vi "resourcesInquiry.vi"(8 "error in (no error)":errorcluster, 11 "HWController in":refnum<class "HWController.lvclass">) -> (0 "error out":errorcluster, 3 "HWController out":refnum<class "HWController.lvclass">)   [LabVIEW 2011, in "Hardware.lvlib" / "HWControllers.lvlib" / "HWController.lvclass"]
uses:
  HWController.lvclass
  HWController.lvclass/HWController.ctl
  HWControllerEvents/HWControllerEvents.lvclass
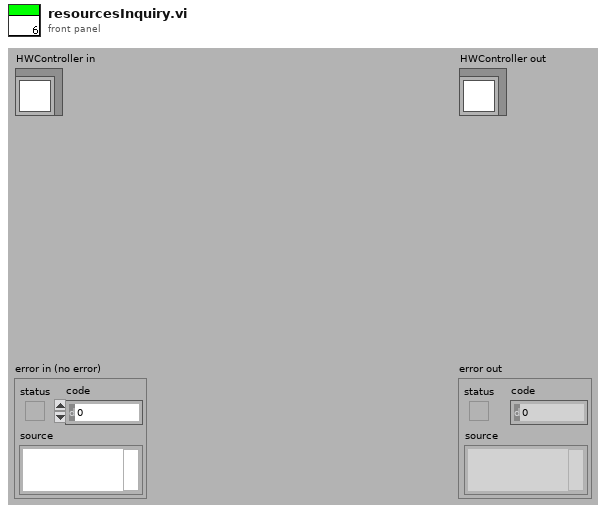
[diagram p1: front panel]
types:
  T1 = enum16{"start", "stop", "statusInquiry", "configure", "resetError", "resourcesInquiry", "reserveResources", "initialise", "resetAllChannels", "staticUpdate", "close", "HWStatus", "error", "resourcesAvailable", "resourcesReserved"}
  T2 = cluster{"incomingEventTypes":cluster{"start":cluster{"Boolean":bool}, "stop":cluster{"Boolean":bool}, "statusInquiry":cluster{"Boolean":bool}, "configure":cluster{"DPScriptPath":path, "TimeStamp":string, "HWLoop?":bool}, "resetError":cluster{"Boolean":bool}, "resourcesInquiry":cluster{"Boolean":bool}, "reserveResources":cluster{"HWList":string[]}, "initialise":cluster{"HWList":string[]}, "close":cluster{"Boolean":bool}, "resetAllChannels":cluster{"Boolean":bool}, "staticChannelUpdate":cluster{"channel_address":string, "calibratedValue":dbl}, "runScript":cluster{"DPScriptPath":path, "TimeStamp":string, "HWLoop?":bool}, "compilingScript":cluster{"Path":path}, "compiledScript":cluster{"Path":path, "timeCompileAt":string}, "compilerError":cluster{"Path":path}, "configureCompiledScript":cluster{"DPScriptPath":path, "TimeStamp":string, "HWLoop?":bool, "CompiledScript":cluster{"ScriptListCompiler.lvclass":refnum<class "ScriptListCompiler.lvclass">, "aoChannels":refnum<class "AnalogOutput.lvclass">[], "doChannels":refnum<class "DigitalOutput.lvclass">[], "rfChannels":refnum<class "DDSOutput.lvclass">[]}}, "restartCompiler":cluster{"restart":bool}, "staticRfChannelUpdate":cluster{"channel_address":string, "Output":cluster{"Frequency(MHz)":dbl, "Amplitude":dbl, "Phase":dbl, "OutputForm":enum16{"Sine", "Square", "Triangle", "Arbitrary"}}}, "cameraUpdate":cluster{"Camera":string, "Type":string, "settings":path}}, "outgoingEventTypes":cluster{"HWStatus":cluster{"status":enum16{"Ready", "Compiling", "Configured", "Running", "Stopping", "Unresolved Error"}}, "error":cluster{"error out":errorcluster}, "resourcesAvailable":cluster{"availableHWList":string[], "reservedHWList":string[]}, "resourcesReserved":cluster{"reservedHWList":string[]}}}
  T3 = cluster{"availableHWList":string[], "reservedHWList":string[]}
  T4 = cluster{"eventId":enum16{"start", "stop", "statusInquiry", "configure", "resetError", "resourcesInquiry", "reserveResources", "initialise", "resetAllChannels", "staticUpdate", "close", "HWStatus", "error", "resourcesAvailable", "resourcesReserved"}, "resourcesAvailable":cluster{"availableHWList":string[], "reservedHWList":string[]}}
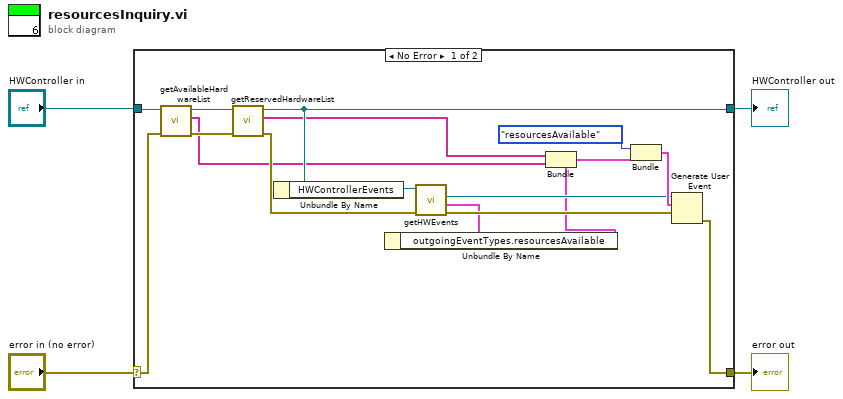
[diagram p0: block diagram]
diagram:
  n1 = case shown="No Error" "error in (no error)" {
    selector: "error in (no error)" -> [w18 w23]
    tunnel: [w8 w23] -> w3
    tunnel: [w17 w22] -> w1
    tunnel: "HWController in" -> [w21 w22]
    frame No Error {
      n2 = call "getAvailableHardwareList.vi"("error in (no error)"=w18, "HWController.lvclass in"=w21) -> ("error out"=w19:errorcluster, "AvailableHardwareList"=w11:string[], "HWController.lvclass out"=w20:refnum<class "HWController.lvclass">)  [unwired: 7 in]
      n3 = call "getReservedHardwareList.vi"("error in (no error)"=w19, "HWController.lvclass in"=w20) -> ("error out"=w15:errorcluster, "reservedHardwareList"=w12:string[], "HWController.lvclass out"=w17:refnum<class "HWController.lvclass">)  [unwired: 7 in]
      n4 = Unbundle By Name(w17) -> ("HWControllerEvents"=w16:refnum<class "HWControllerEvents.lvclass">)
      n5 = call-dynamic "getHWEvents.vi"("error in (no error)"=w15, "HWControllerEvents in"=w16) -> ("error out"=w9:errorcluster, "eventDataTypes"=w7:T2, "HWCEvent"=w13:refnum<user-event>)  [unwired: 6 in, 1 out]
      n6 = Unbundle By Name(w7) -> ("outgoingEventTypes.resourcesAvailable"=w6:T3)
      n7 = Bundle(cluster=w6, "availableHWList"=w12, "reservedHWList"=w11) -> (w10:T3)
      n8 = Bundle("eventId"=T1."resourcesAvailable", "resourcesAvailable"=w10) -> (w14:T4)  [unwired: 1 in]
      n9 = Generate User Event(user event=w13, event data cluster=w14, error in=w9) -> (error out=w8:errorcluster)  [unwired: 1 out]
    }
    frame Error {
    }
  }
  "error out" <- w3
  "HWController out" <- w1
